vi "Command (read & write) - SP.vi"(7 "timeout ms (100)":i32=100, 8 "error in (no error)":errorcluster, 9 "Position":i32=-2147483648, 10 "IP":string, 11 "connection ID in":refnum<k16>) -> (0 "error out":errorcluster, 2 "Position":i32, 3 "connection ID out":refnum<k16>)   [LabVIEW 2016, in "SMD-7615.lvlib" / "eSCL.lvlib"]
doc: "SP - Set Position\nSets or requests the motor’s absolute position. To ensure that the internal position counter resets properly, use EP immediately prior to sending SP. For example, to set the position to zero after a homing routine, send EP0 immediately followed by SP0."
uses:
  eSCL.lvlib
  I32 Command and Param.ctl
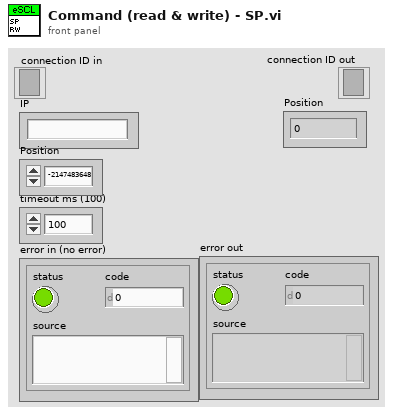
[diagram p1: front panel]
types:
  T1 = typedef "SMD-7615.lvlib/eSCL.lvlib/I32 Command and Param.ctl" = cluster{"Command":string, "I32 Parameler":i32, "I32 Parameler Default":i32, "I32 Parameler Coerece Upper":i32, "I32 Parameler Coerece Lower":i32}
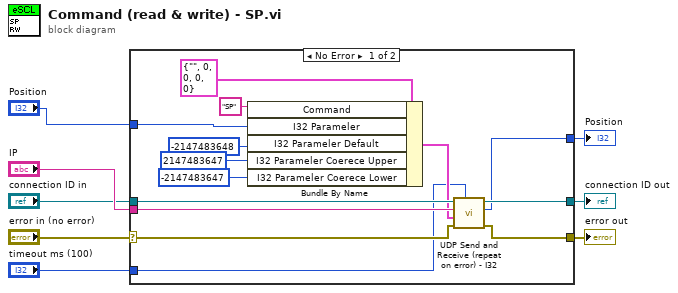
[diagram p0: block diagram]
diagram:
  n1 = case shown="No Error" "error in (no error)" {
    selector: "error in (no error)" -> [w14 w23]
    tunnel: "connection ID in" -> [w17 w24]
    tunnel: [w12 w24] -> w3
    tunnel: [w11 w23] -> w2
    tunnel: "IP" -> [w16 _]
    tunnel: "timeout ms (100)" -> [w13 _]
    tunnel: "Position" -> [w18 _]
    tunnel: [w9 _] -> w1
    frame No Error {
      n2 = Bundle By Name(cluster=T1 {"Command"="", "I32 Parameler"=0, "I32 Parameler Default"=0, "I32 Parameler Coerece Upper"=0, "I32 Parameler Coerece Lower"=0} ("I32 Command & Param"), "Command"="SP", "I32 Parameler"=w18, "I32 Parameler Default"=-2147483648 ("DBL Parameler Default"), "I32 Parameler Coerece Upper"=2147483647 ("DBL Parameler Coerece Upper"), "I32 Parameler Coerece Lower"=-2147483647 ("DBL Parameler Coerece Lower")) -> (w15:T1)
      n3 = call "UDP Send and Receive (repeat on error) - I32.vi"("timeout ms (100)"=w13, "error in (no error)"=w14, "I32 Command & Param"=w15, "IP"=w16, "connection ID in"=w17) -> ("error out"=w11:errorcluster, "I32 Param out"=w9:i32, "connection ID out"=w12:refnum<k16>)  [unwired: 4 in]
    }
    frame Error {
    }
  }
  "connection ID out" <- w3
  "error out" <- w2
  "Position" <- w1
